vi "InitEditor.vi"(8 "error in (no error)":errorcluster {"code" format="Error %.0f"}, 10 "VIDoc Settings Path":path, 11 "VIDoc Settings In":refnum<class "VIDoc Settings.lvclass">) -> (0 "error out":errorcluster {"code" format="Error %.0f"}, 3 "VIDoc Settings Out":refnum<class "VIDoc Settings.lvclass">)   [LabVIEW 2023, in "VIDoc Settings.lvclass"]
uses:
  VIDoc Settings.lvclass
  VIDoc Settings.lvclass/VIDoc Settings.ctl
  Set VIDoc Settings Path.vi
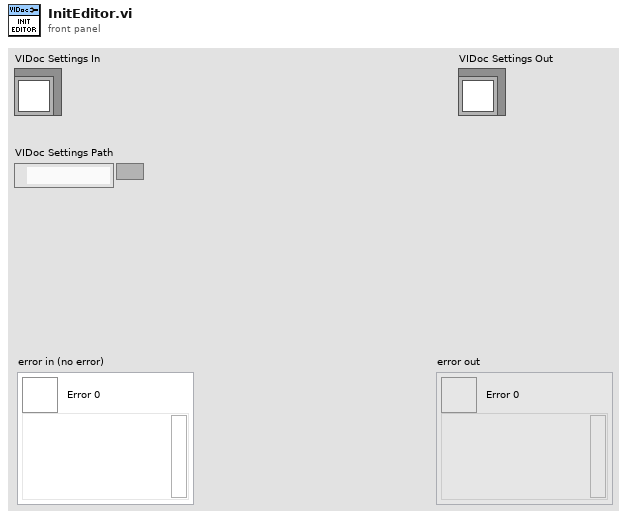
[diagram p1: front panel]
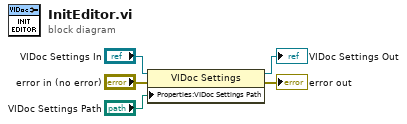
[diagram p0: block diagram]
diagram:
  n1 = property class="VIDoc Settings"(reference="VIDoc Settings In", error in="error in (no error)", "Properties:VIDoc Settings Path"="VIDoc Settings Path") -> (reference out=→"VIDoc Settings Out":refnum<class "VIDoc Settings.lvclass">, error out=→"error out":errorcluster)
